vi "MeasuringDevice.GetMeasurementResult.vi"(8 "error in (no error)":errorcluster, 9 "Count (1)":i32=1, 10 "Offset (0)":i32, 11 "MeasuringDevice":refnum<class "MeasuringDevice.lvclass">) -> (0 "error out":errorcluster, 2 "Result":variant[](array[variant]), 3 "MeasuringDevice out":refnum<class "MeasuringDevice.lvclass">)   [LabVIEW 2017, in "MeasuringDevice.lvclass"]
doc: "---------------------------------------------------------------\nJKI State Machine Objects™\nhttp://jki.net/state-machine-objects/\nCopyright (C) 2005-2015, JKI <info@jki.net>\nALL RIGHTS RESERVEDJKI State Machine Objects (SMO) 1.0.0.5\nJKI - JKI\nCopyright (c) 2016, JKI"
uses:
  MeasuringDevice.lvclass
  CircularBuffer/CircularBuffer.lvclass
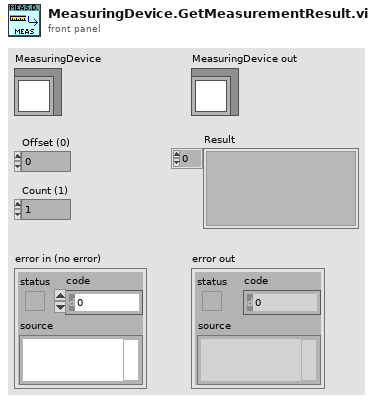
[diagram p1: front panel]
types:
  T1 = typedef "MeasuringDevice.lvclass/Dependencies--Cluster.ctl" = cluster{"MeasurementBuffer":refnum<class "CircularBuffer.lvclass">}
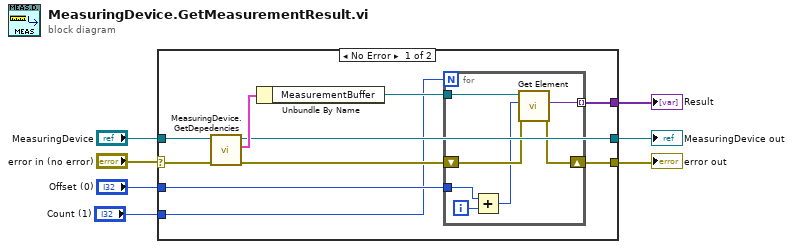
[diagram p0: block diagram]
diagram:
  n1 = case shown="No Error" "error in (no error)" {
    selector: "error in (no error)" -> [w16 w25]
    tunnel: "MeasuringDevice" -> [w17 w26]
    tunnel: [w11 w26] -> w6
    tunnel: [w10 w25] -> w4
    tunnel: "Offset (0)" -> [w9 _]
    tunnel: [w12 _] -> w2
    tunnel: "Count (1)" -> [w8 _]
    frame No Error {
      n2 = call "MeasuringDevice.GetDepedencies.vi"("error in (no error)"=w16, "MeasuringDevice"=w17) -> ("error out"=w13:errorcluster, "Dependencies"=w15:T1, "MeasuringDevice"=w11:refnum<class "MeasuringDevice.lvclass">)  [unwired: 7 in]
      n3 = Unbundle By Name(w15) -> ("MeasurementBuffer"=w14:refnum<class "CircularBuffer.lvclass">)
      n4 = for {
        N: w8 -> [_]
        tunnel: w14 -> [w24]
        tunnel: [w22] -> w12 mode=indexing
        shift-right: [w21] -> w10
        shift-left: w13 -> [w23]
        tunnel: w9 -> [w19]
        i -> [w20]
        n5 = Add(x=w19, y=w20) -> (x+y=w18:i32)
        n6 = call "Get Element.vi"("error in (no error)"=w23, "GetElement (-1: Current)"=w18, "CircularBuffer"=w24) -> ("error out"=w21:errorcluster, "Element"=w22:variant)  [unwired: 6 in, 1 out]
      }
    }
    frame Error {
    }
  }
  "error out" <- w4
  "MeasuringDevice out" <- w6
  "Result" <- w2
